vi "initArduinoNew.vi"(0 "VISA resource":refnum<visa-resource-name>="COM3") -> ()   [LabVIEW 2012]
uses:
  <vilib>/LabVIEW Interface for Arduino/Type Defs/Pin Mode.ctl
  GlobalArduinoNew.vi
  <vilib>/LabVIEW Interface for Arduino/LabVIEW Interface for Arduino.lvlib
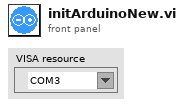
[diagram p1: front panel]
types:
  T1 = typedef "LabVIEW Interface for Arduino.lvlib/Pin Mode.ctl" = enum8{"Input", "Output"}
  T2 = typedef "LabVIEW Interface for Arduino.lvlib/Arduino Resource.ctl" = cluster{"VISA resource":refnum<visa-resource-name>, "Board Type":T3, "Connection Type":enum8{"USB / Serial"}, "Bytes Per Packet (15)":u8}
  T3 = typedef "LabVIEW Interface for Arduino.lvlib/Board Type.ctl" = enum16{"Uno", "Dimuelanove w/Atmega 328", "Mega 2560"}
  T4 = typedef "Semaphore RefNum" = refnum<k1>
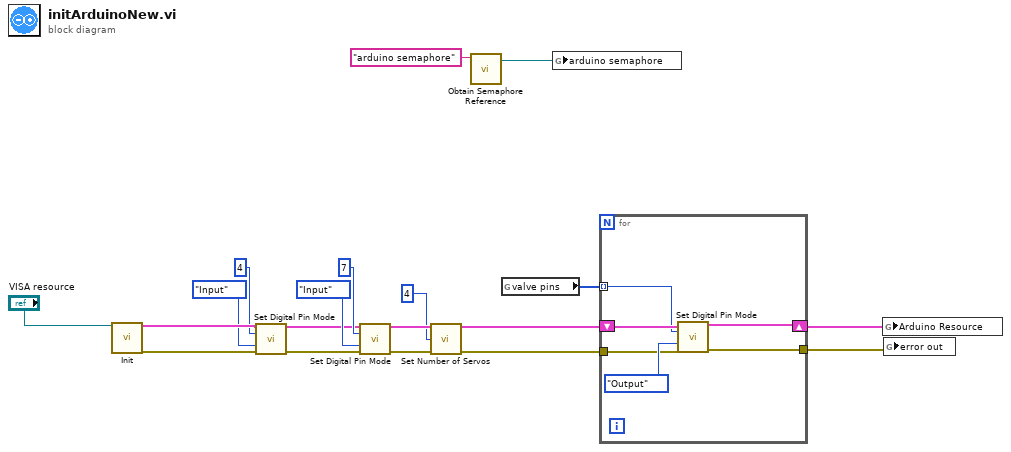
[diagram p0: block diagram]
diagram:
  n1 = call <vilib>:"Init.vi"("VISA resource"="VISA resource") -> ("Arduino Resource"=w18:T2, "error out"=w17:errorcluster)  [unwired: 17 in]
  n2 = call <vilib>:"Set Digital Pin Mode.vi"("Arduino Resource"=w18, "Digital I/O Pin"=u8 4, "Pin Mode (Input)"=Pin_Mode."Input", "error in"=w17) -> ("Arduino Resource"=w12:T2, "error out"=w11:errorcluster)  [unwired: 10 in]
  n3 = call <vilib>:"Set Digital Pin Mode.vi"("Arduino Resource"=w12, "Digital I/O Pin"=u8 7, "Pin Mode (Input)"=Pin_Mode."Input", "error in"=w11) -> ("Arduino Resource"=w9:T2, "error out"=w10:errorcluster)  [unwired: 10 in]
  n4 = call <vilib>:"Set Number of Servos.vi"("Arduino Resource"=w9, "Number Of Servos (1)"=u8 4, "error in"=w10) -> ("Arduino Resource"=w6:T2, "error out"=w4:errorcluster)  [unwired: 11 in]
  n5 = call <vilib>:"Obtain Semaphore Reference.vi"("name (unnamed)"="arduino semaphore") -> ("semaphore"=w2:T4)  [unwired: 4 in, 2 out]
  n6 = global read "GlobalArduinoNew.vi" "valve pins"() -> (w7:u8[])
  n7 = global write "GlobalArduinoNew.vi" "arduino semaphore"(w2) -> ()
  n8 = for {
    tunnel: w7 -> [w23] mode=indexing
    shift-right: [w24] -> w5
    shift-left: w6 -> [w25]
    tunnel: w4 -> [w21]
    tunnel: [w20] -> w3
    n9 = call <vilib>:"Set Digital Pin Mode.vi"("Arduino Resource"=w25, "Digital I/O Pin"=w23, "Pin Mode (Input)"=Pin_Mode."Output", "error in"=w21) -> ("Arduino Resource"=w24:T2, "error out"=w20:errorcluster)  [unwired: 10 in]
  }
  n10 = global write "GlobalArduinoNew.vi" "Arduino Resource"(w5) -> ()
  n11 = global write "GlobalArduinoNew.vi" "error out"(w3) -> ()
